vi "TDM Transfer Receive Simulation.vi"() -> ()   [LabVIEW 2013]
uses:
  <vilib>/rvi/DesktopExecutionNode/Execution/niFpgaDEN_Execute.vi
  <vilib>/rvi/DesktopExecutionNode/DesktopExecutionNode.xnode
  Source/I2S-TDM.lvlib
panel:
  out "sample in":u32
  out "Samples Read":u32[](array[numeric])
  in  "Loop Wait":u32(slide)=45 min=10 max=70 step=1 scale=10.0..70.0
  in  "channel count":u8=2
  in  "transmit":bool
  in  "pause":bool
  in  "24-bit data":bool[](array[boolean])=[TRUE, FALSE, FALSE, TRUE, TRUE, FALSE, FALSE, TRUE, FALSE, TRUE, FALSE, FALSE, FALSE, FALSE, FALSE, FALSE, FALSE, FALSE, FALSE, FALSE, FALSE, FALSE, FALSE, TRUE]
  out "Digital Waveform Graph":digitalwaveform(graph)
  in  "bits per channel":u8=32
  in  "stop":bool
  # "MSB"
  # "LSB"
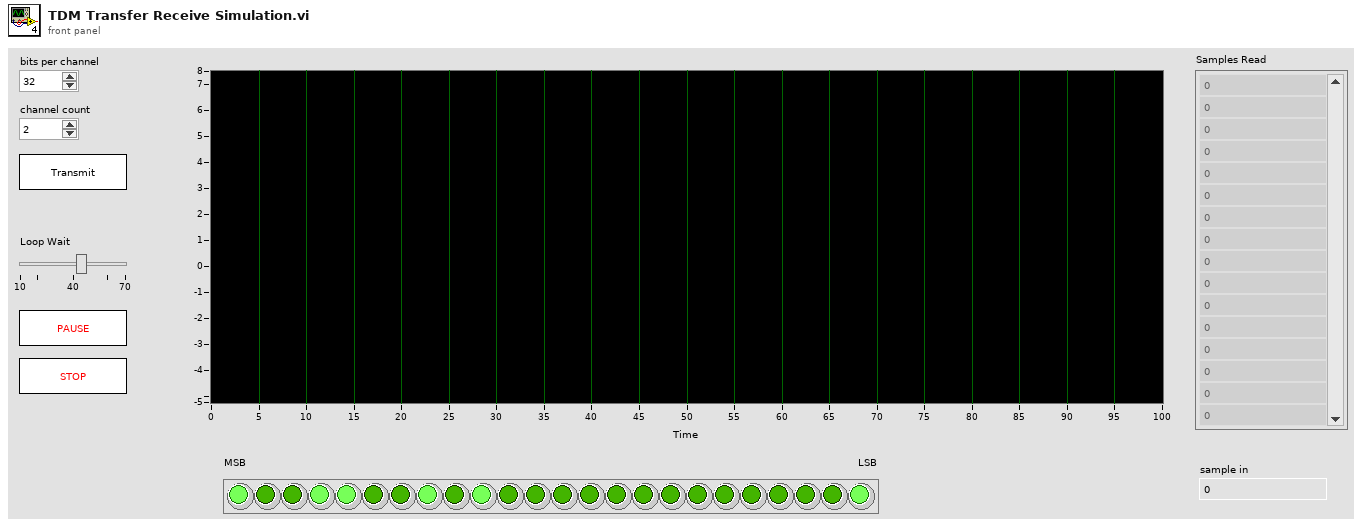
[diagram p1: front panel]
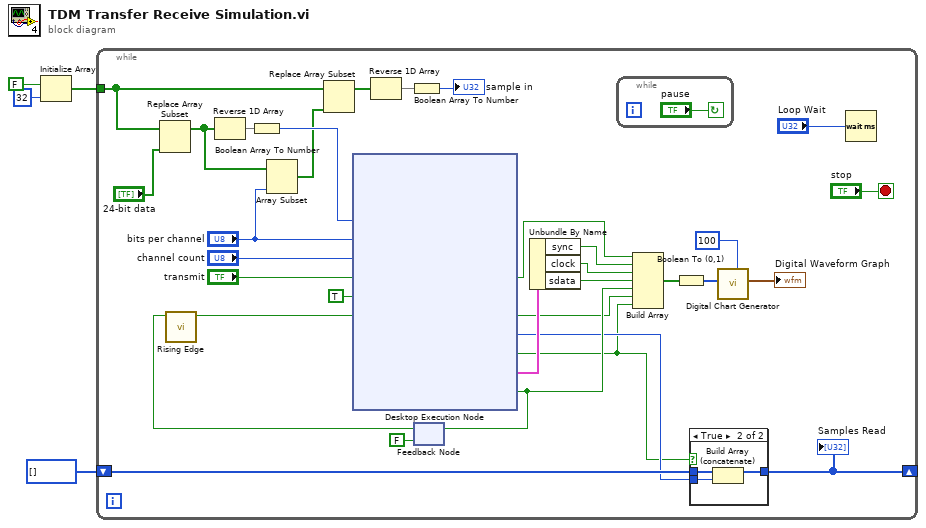
[diagram p0: block diagram]
diagram:
  n1 = Initialize Array(FALSE, 32 ("dimension size")) -> (w2:bool[])
  n2 = while {
    tunnel: w2 -> [w7]
    shift-right: [w15] -> _
    shift-left: u32[] [] -> [w17]
    stop <- "stop" stop-if-true
    n3 = Replace Array Subset(array=w7, new element="24-bit data") -> (w8:bool[])  [unwired: 1 in]
    n4 = Reverse 1D Array(array=w8) -> (reversed array=w34:bool[])
    n5 = Boolean Array To Number(Boolean array=w34) -> (number=w29:u32)
    n6 = Array Subset(array=w8, length="bits per channel") -> (w6:bool[])  [unwired: 1 in]
    n7 = Replace Array Subset(array=w7, new element=w6) -> (w5:bool[])  [unwired: 1 in]
    n8 = Reverse 1D Array(array=w5) -> (reversed array=w11:bool[])
    n9 = Boolean Array To Number(Boolean array=w11) -> (number=→"sample in":u32)
    n10 = feedback #1(FALSE ("ready for input")) -> (w31:bool)
    n11 = call "Rising Edge.vi"("signal in"=w31) -> ("rising edge?"=w30:bool)  [unwired: 10 in]
    n12 = xnode "Desktop Execution Node"("sample in"=w29, "transfer length"="bits per channel", "channel count"="channel count", "transfer"="transmit", "ready for output"=TRUE, "input valid"=w30) -> ("transfer"=w13:bool, "input valid"=w18:bool, "sample out"=w16:u32, "output valid"=w14:bool, "signals out"=w25:cluster{"clock":bool, "sync":bool, "sdata":bool}, "ready for input"=w19:bool)  [unwired: 1 in, 1 out]
    n13 = feedback-in #1(w19) -> ()
    n14 = Unbundle By Name(w25) -> ("sync"=w24:bool, "clock"=w23:bool, "sdata"=w22:bool)
    n15 = while {
      stop <- "pause" continue-if-true
    }
    n16 = Build Array(w13, w24, w23, w22, w19, w18, w14) -> (w21:bool[])
    n17 = Boolean To (0,1)(Boolean=w21) -> (0, 1=w20:i16[])
    n18 = case shown="True" w14 {
      tunnel: w17 -> [w38 w41]
      tunnel: w16 -> [_ w40]
      tunnel: [w38 w39] -> w15
      frame False {
      }
      frame True {
        n19 = Build Array (concatenate)(w41, w40) -> (w39:u32[])
      }
    }
    "Samples Read" <- w15
    n20 = call "Digital Chart Generator.vi"("History Size"=100, "Input"=w20) -> ("Digital Data"=→"Digital Waveform Graph":digitalwaveform)  [unwired: 9 in]
    n21 = Wait (ms)(milliseconds to wait="Loop Wait") -> ()  [unwired: 1 out]
  }
